vi "Reset and Start Test.vi"(7 "Tx/Rx":T2=enum."Rx", 8 "error in (no error)":errorcluster, 9 "Tx Packet Type":T1, 10 "BLE Channel Number (0-39)":u8, 11 "VISA Refnum in":refnum<visa-resource-name>) -> (0 "error out":errorcluster, 2 "Array":string[](array[string]), 3 "VISA Refnum out":refnum<visa-resource-name>)   [LabVIEW 2026, in "Nordic nRF52 DK DTM Test.lvlib"]
uses:
  Nordic nRF52 DK DTM Test.lvlib
  TxRx.ctl
  PacketType.ctl
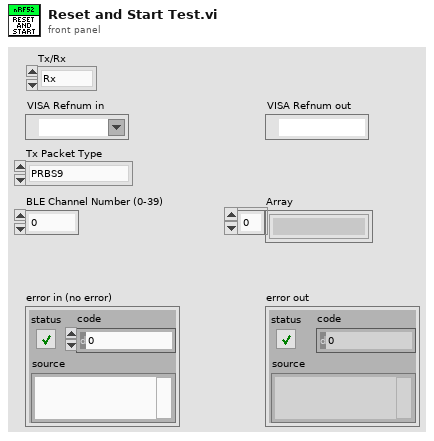
[diagram p1: front panel]
types:
  T1 = typedef "Nordic nRF52 DK DTM Test.lvlib/PacketType.ctl" = enum16{"PRBS9", "DF1", "DF2"}
  T2 = typedef "Nordic nRF52 DK DTM Test.lvlib/TxRx.ctl" = enum16{"Tx", "Rx"}
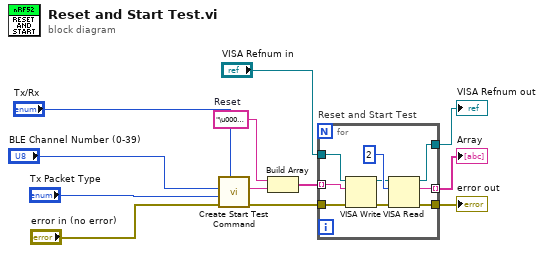
[diagram p0: block diagram]
diagram:
  w9 = "\u0000\u0000"  # Reset
  n1 = call "Create Start Test Command.vi"("Tx/Rx"="Tx/Rx", "error in (no error)"="error in (no error)", "Tx Packet Type"="Tx Packet Type", "BLE  Channel (Decimal)"="BLE Channel Number (0-39)") -> ("error out"=w12:errorcluster, "VISA Hex Cmd"=w6:string)  [unwired: 6 in]
  n2 = Build Array(w9, w6) -> (w10:string[])
  n3 = for "Reset and Start Test" {
    tunnel: w12 -> [w21]
    tunnel: "VISA Refnum in" -> [w20]
    tunnel: [w16] -> w3
    tunnel: [w15] -> w4
    tunnel: [w14] -> w5 mode=indexing
    tunnel: w10 -> [w13] mode=indexing
    n4 = VISA Write(VISA resource name=w20, write buffer=w13, error in (no error)=w21) -> (VISA resource name out=w17:refnum<visa-resource-name>, error out=w18:errorcluster)  [unwired: 1 out]
    n5 = VISA Read(VISA resource name=w17, byte count=u32 2, error in (no error)=w18) -> (VISA resource name out=w16:refnum<visa-resource-name>, read buffer=w14:string, error out=w15:errorcluster)  [unwired: 1 out]
  }
  "Array" <- w5
  "error out" <- w4
  "VISA Refnum out" <- w3
